vi "FTW-Test-JSON-DAQ-Types.vi"() -> ()   [LabVIEW 2015]
uses:
  source/Reflection/FTW-Reflection-Types.ctl
  <vilib>/Utility/Data Type/Type Definitions/Data Type.ctl
  <vilib>/Utility/Data Type/NI_Data Type.lvlib
panel:
  out "Array":T1[](array[typedef])
  out "Cluster Elements":T3(array[cluster])
  out "JSON String":string
  out "data":T4
  in  "DAQmx Terminal":tag
  in  "DAQmx Task Name":refnum<k21>
  in  "DAQmx Switch":tag
  in  "DAQmx Scale Name":tag
  in  "DAQmx Physical Channel":tag
  in  "DAQmx Global Channel":refnum<k21>
  in  "DAQmx Device Name":tag
  out "error out":errorcluster
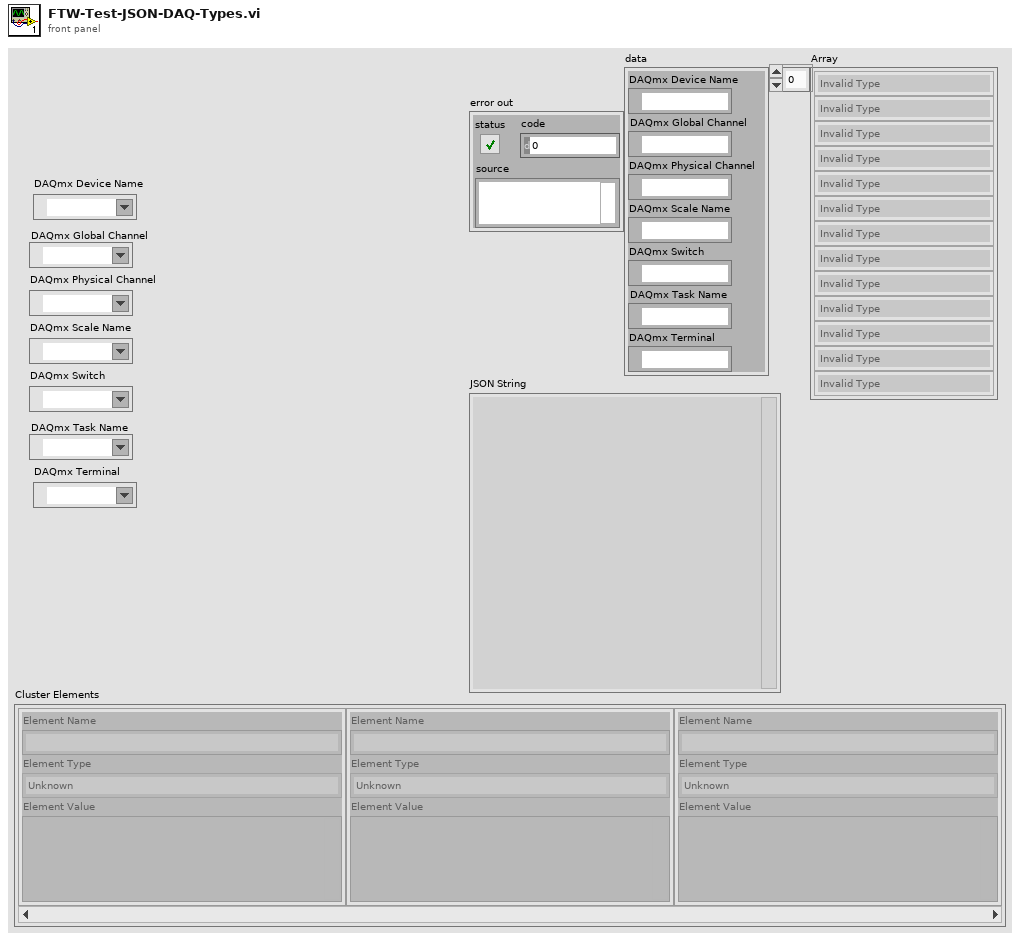
[diagram p1: front panel]
types:
  T1 = typedef "NI_Data Type.lvlib/Data Type.ctl" = enum8{"Invalid Type", "Void", "I8", "I16", "I32", "I64", "U8", "U16", "U32", "U64", "Single Float", "Double Float", "Extended Float", "Single Complex", "Double Complex", "Extended Complex", "Enum U8", "Enum U16", "Enum U32", "Enum U64", "Single Float With Unit", "Double Float With Unit", "Extended Float With Unit", "Single Complex with Unit", "Double Complex with Unit", "Extended Complex with Unit", "Boolean", "String", "Path", "Picture", "Tag", "Array", "Cluster", "Variant", "LV Variant", "Waveform", "Timestamp", "Digital Waveform", "Digital Data", "ExpressData", "Refnum", "External Data", "VI", "Poly VI", "LabVIEW Class Instance", "Fixed Point"}
  T2 = typedef "FTW-Reflection-Types.ctl" = enum16{"Unknown", "Void", "Array", "Cluster", "LVObject", "Boolean", "I8", "I16", "I32", "I64", "U8", "U16", "U32", "U64", "SGL", "DBL", "EXT", "CSG", "CDB", "CXT", "FXP", "EnumU8", "EnumU16", "EnumU32", "EnumU64", "SGLwithUnit", "DBLwithUnit", "EXTwithUnit", "CSGwithUnit", "CDBwithUnit", "CXTwithUnit", "String", "Path", "Picture", "Tag", "LVVariant", "Timestamp", "WaveformI8", "WaveformI16", "WaveformI32", "WaveformI64", "WaveformU8", "WaveformU16", "WaveformU32", "WaveformU64", "WaveformSGL", "WaveformDBL", "WaveformEXT", "WaveformCSG", "WaveformCDB", "WaveformCXT", "WaveformDigital", "WaveformUnknownType", "DigitalData", "DynamicData", "ExternalData", "FileByteStream", "TDMStream", "dotNET", "ActiveX", "VIServerReference", "VIReference", "ApplicationInstance", "Menu", "ConnectionDataSocket", "ConnectionVISA", "ConnectionBluetooth", "ConnectionIrDA", "ConnectionTCP", "ConnectionUDP", "ConnectionHTTPClient", "ConnectionFTP", "Occurrence", "Notifier", "Queue", "Rendezvous", "Semaphore", "RTFIFO", "EventPublisher", "EventRegistration", "EventCallback", "DataValueReference", "GenericClass", "GenericClassTag", "GenericClassDeepCopy", "GenericClassFlattened", "GenericClassTagFlattened", "GenericReferenceType", "WindowsRegistry", "OverloadedDatalogRef", "ReferenceUnknownType"}
  T3 = cluster{"Element Name":string, "Element Type":T2, "Element Value":variant}[]
  T4 = cluster{"DAQmx Device Name":tag, "DAQmx Global Channel":refnum<k21>, "DAQmx Physical Channel":tag, "DAQmx Scale Name":tag, "DAQmx Switch":tag, "DAQmx Task Name":refnum<k21>, "DAQmx Terminal":tag}
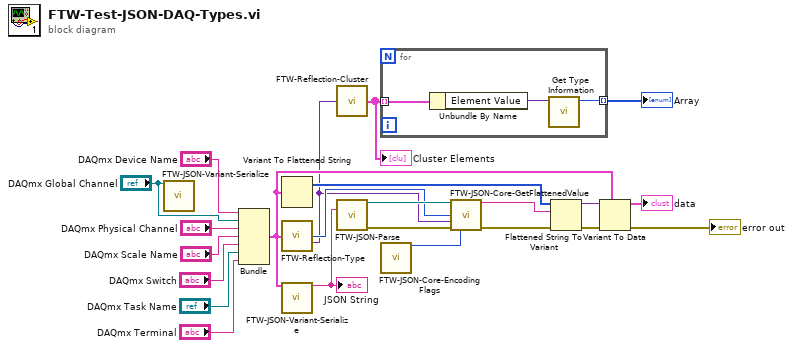
[diagram p0: block diagram]
diagram:
  n1 = call "FTW-JSON-Variant-Serialize.vi"("Variant"="DAQmx Global Channel") -> ()  [unwired: 13 in, 2 out]
  n2 = Bundle("DAQmx Device Name"="DAQmx Device Name", "DAQmx Global Channel"="DAQmx Global Channel", "DAQmx Physical Channel"="DAQmx Physical Channel", "DAQmx Scale Name"="DAQmx Scale Name", "DAQmx Switch"="DAQmx Switch", "DAQmx Task Name"="DAQmx Task Name", "DAQmx Terminal"="DAQmx Terminal") -> (w6:T4)  [unwired: 1 in]
  n3 = Variant To Flattened String(Variant=w6) -> (1:w22:i16[])  [unwired: 1 out]
  n4 = call "FTW-Reflection-Type.vi"("Anything"=w6) -> ("LabVIEW Type"=w16:T2, "Variant Type and Value"=w4:variant)  [unwired: 12 in, 1 out]
  n5 = call "FTW-JSON-Variant-Serialize.vi"("Variant"=w6) -> ("JSON String"=w5:string)  [unwired: 13 in, 1 out]
  "JSON String" <- w5
  n6 = call "FTW-Reflection-Cluster.vi"("Cluster"=w4) -> ("Cluster Elements"=w3:T3)  [unwired: 14 in]
  "Cluster Elements" <- w3
  n7 = call "FTW-JSON-Parse.vi"("JSON String"=w5) -> ("Container"=w18:refnum<class "FTW-Container.lvclass">, "error out"=w15:errorcluster)  [unwired: 13 in]
  n8 = for {
    tunnel: w3 -> [w26] mode=indexing
    tunnel: [w24] -> w2 mode=indexing
    n9 = Unbundle By Name(w26) -> ("Element Value"=w25:variant)
    n10 = call <vilib>:"Get Type Information.vi"("Variant"=w25) -> ("Type"=w24:T1)  [unwired: 6 in, 4 out]
  }
  "Array" <- w2
  n11 = call "FTW-JSON-Core-EncodingFlags.vi"() -> ("Encoding Flags"=w17:i64)  [unwired: 14 in, 1 out]
  n12 = call "FTW-JSON-Core-GetFlattenedValue.vi"("Container"=w18, "LabVIEW Type"=w16, "Element Default Value"=w4, "error in"=w15, "Encoding Flags"=w17) -> ("Flattened Value"=w21:string, "error out"=w19:errorcluster)  [unwired: 9 in]
  n13 = Flattened String To Variant(4:w19, 6:w21, 7:w22) -> (0:w20:errorcluster, 3:w23:variant)
  n14 = Variant To Data(error in=w20, type=w6, Variant=w23) -> (data=→"data":T4, error out=→"error out":errorcluster)
